vi "DataLoggerModule.vi"(8 "error in (no error)":errorcluster, 9 "Shutdown Event":refnum<user-event>, 10 "Config":cluster{"Tag List":string[]}, 11 "ModuleID":string) -> (0 "error out":errorcluster)   [LabVIEW 2020, in "DataLogger.lvlib"]
uses:
  DataLogger.lvlib
  <vilib>/Tag Engine/Tag/Tag.lvclass
  <vilib>/Tag Engine/Types/SetRequest Cluster.ctl
  <vilib>/Utility/Data Type/Type Definitions/Data Type.ctl
  <vilib>/Tag Engine/Tag/Tag.lvclass/Tag.ctl
  80db7cca-9c65-475a-8561-7a2b6cce7442.vi
  df08592d-67de-40ba-a6cc-0fa837fd12aa.vi
  f9099f2b-b695-4638-8a60-8ed48ec280e8.vi
  5108da9f-c4b3-4642-ad75-afbb112a1f2a.vi
  c28e23b0-67fd-4dd8-8582-f417e2518810.vi
  2954e155-24bd-4d8b-b20f-9ca0e37c8e83.vi
  <vilib>/Tag Engine/Tag/Read Name.vi
  <vilib>/Tag Engine/Tag/Read Units.vi
  <vilib>/Tag Engine/API/Get Tag SetRequest Event.vi
  <vilib>/Tag Engine/Tools/SubVIs/Array of VData to VCluster_openG.vi
  <vilib>/Tag Engine/API/Get Tag Value_ByRef.vi
  <vilib>/Tag Engine/API/Write Tag Value_ByRef.vi
  <vilib>/Tag Engine/Tag/Read SetRequest Event.vi
  <vilib>/Tag Engine/Tag/Read Value.vi
  <vilib>/Tag Engine/Tag/Read Timestamp.vi
  <vilib>/Tag Engine/Tag/Write Value with Timestamp.vi
  <vilib>/Utility/Data Type/Get Type Information.vi
  <vilib>/JDP Science/JSONtext/Variant to JSON Text.vi
  <vilib>/Tag Engine/Core/Tag Lookup_By Name.vi
  <vilib>/Utility/Data Type/Get Cluster Information.vi
  <vilib>/Utility/Data Type/NI_Data Type.lvlib
  <vilib>/Tag Engine/Tag Engine Core.lvlib
  <vilib>/Tag Engine/Tag Engine.lvlib
  1b9bca86-45d1-4ef5-b749-ac0dbadf3a5e.vi
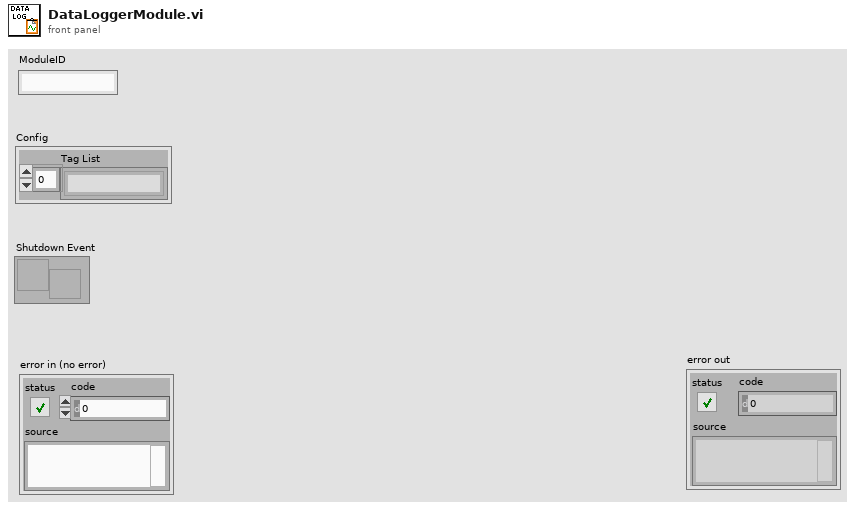
[diagram p1: front panel]
types:
  T1 = cluster{"LOG_EN":refnum<user-event>, "FILE":refnum<user-event>, "PERIOD":refnum<user-event>}
  T2 = cluster{"Tag Refs":cluster{"LOG_EN":refnum<data-value>, "FILE":refnum<data-value>, "PERIOD":refnum<data-value>}, "Config":cluster{"Tag List":string[]}, "LogTagRefs":refnum<data-value>[], "Period":i32, "En":bool, "FileRef":refnum<file>, "FilePath":path}
  T3 = cluster{"LOG_EN":refnum<data-value>, "FILE":refnum<data-value>, "PERIOD":refnum<data-value>}
  T4 = cluster{"Req Value":i32, "Callback":refnum<notifier>}
  T5 = cluster{"Req Value":path, "Callback":refnum<notifier>}
  T6 = enum16{"open", "replace", "create", "open or create", "replace or create", "replace or create with confirmation"}
  T7 = cluster{"Req Value":variant, "Callback":refnum<notifier>}
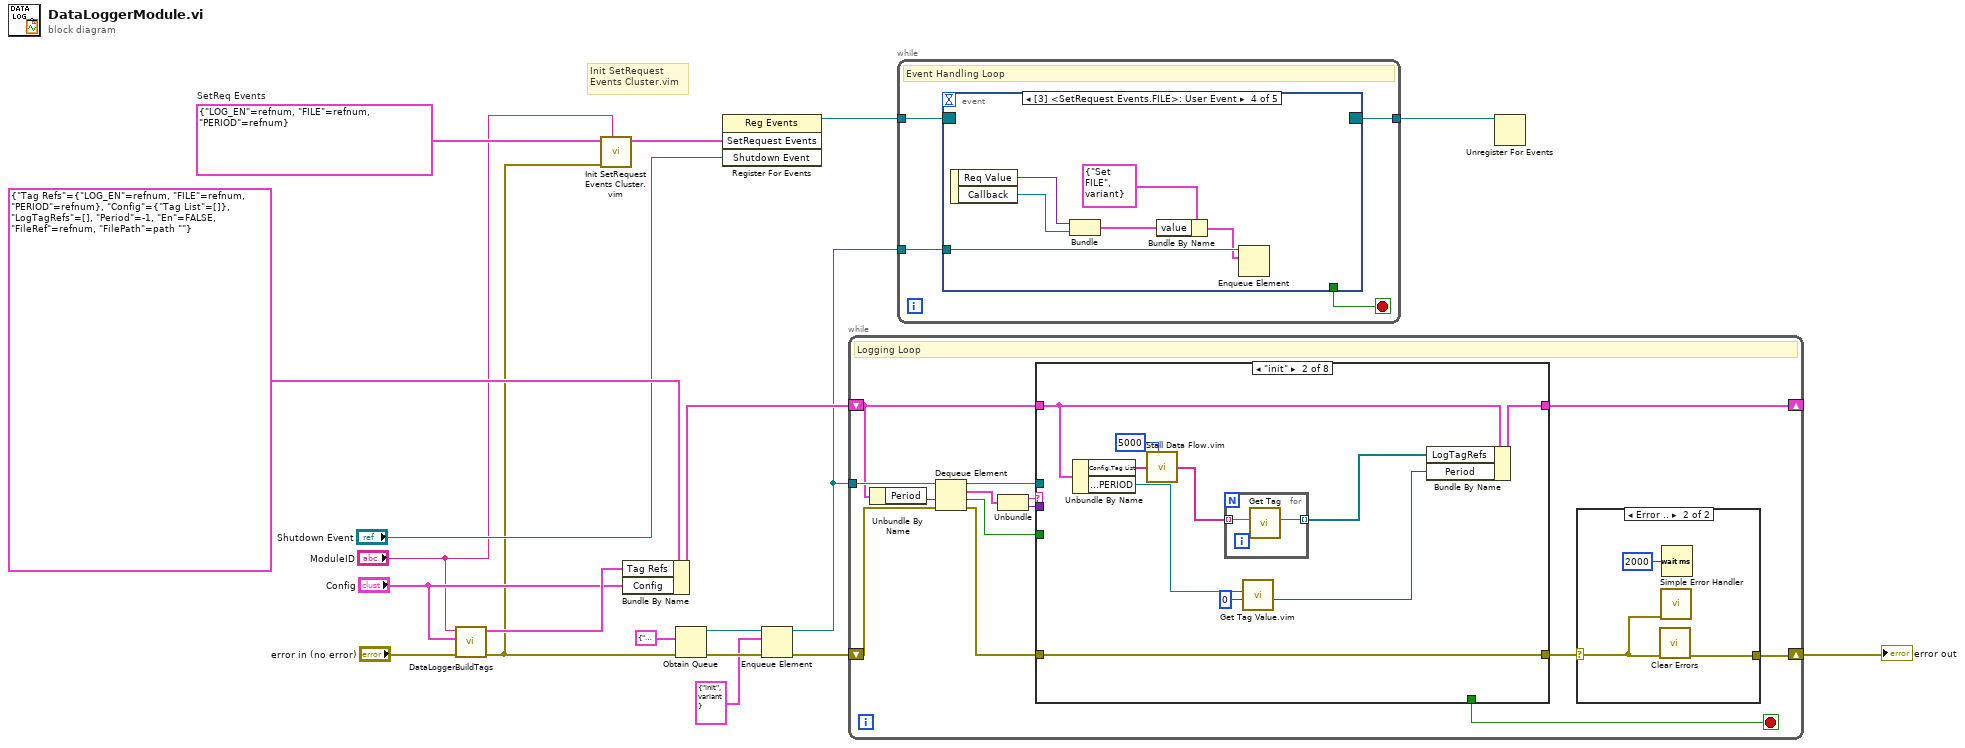
[diagram p0: block diagram]
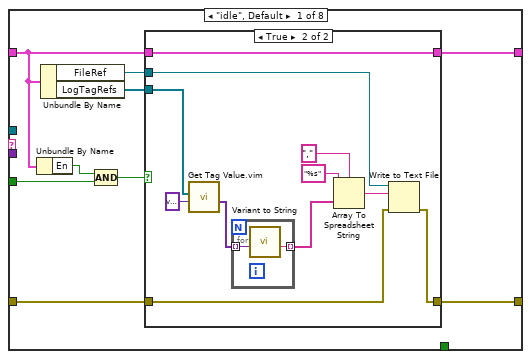
[diagram p3: hidden frame]
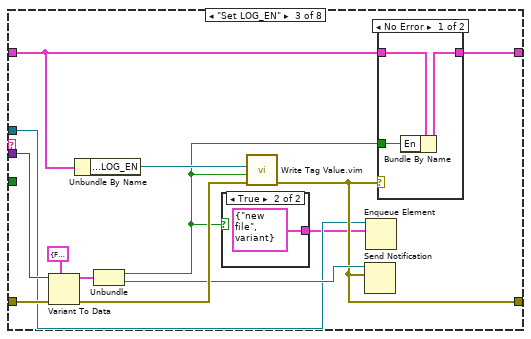
[diagram p5: hidden frame]
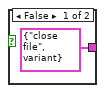
[diagram p6: hidden frame]
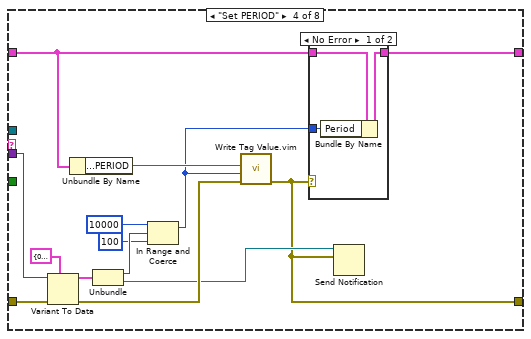
[diagram p8: hidden frame]
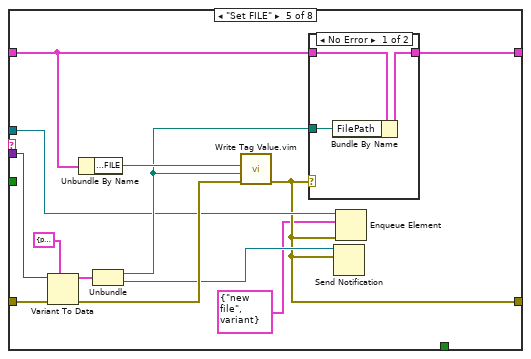
[diagram p10: hidden frame]
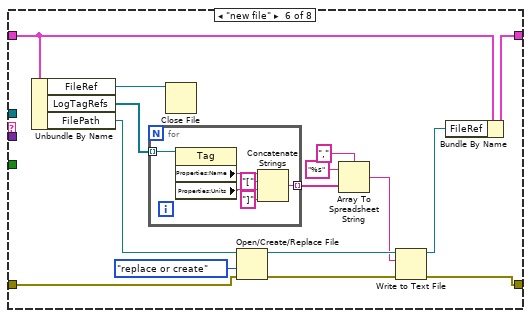
[diagram p12: hidden frame]
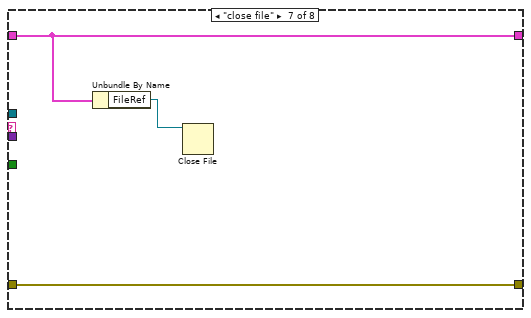
[diagram p13: hidden frame]
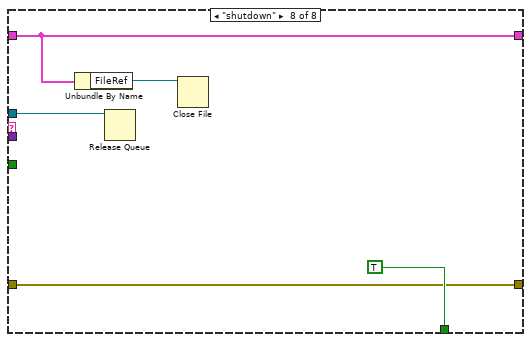
[diagram p14: hidden frame]
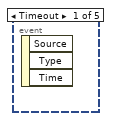
[diagram p15: hidden frame]
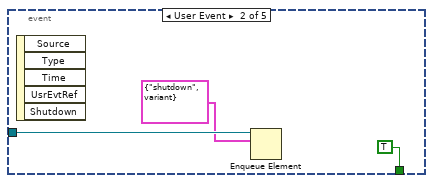
[diagram p16: hidden frame]
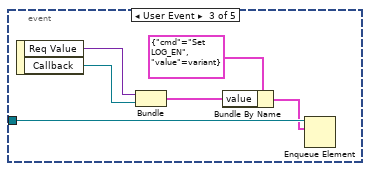
[diagram p17: hidden frame]
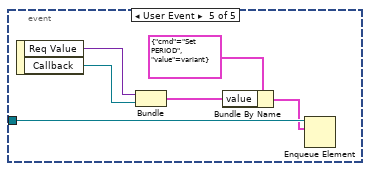
[diagram p18: hidden frame]
diagram:
  w5 = T1 {"LOG_EN"=refnum, "FILE"=refnum, "PERIOD"=refnum}  # SetReq Events
  # "Init SetRequest\nEvents Cluster.vim"
  n1 = call "DataLoggerBuildTags.vi"("error in (no error)"="error in (no error)", "Config"="Config", "ModuleID"="ModuleID") -> ("error out"=w2:errorcluster, "Tag Refs"=w12:T3)  [unwired: 7 in]
  n2 = call "Init SetRequest Events Cluster.vim"("Namespace"="ModuleID", "error in (no error)"=w2, "SetRequest Events in"=w5) -> ("SetRequest Events"=w3:T1)  [unwired: 7 in, 1 out]
  n3 = Bundle By Name(cluster=T2 {"Tag Refs"={"LOG_EN"=refnum, "FILE"=refnum, "PERIOD"=refnum}, "Config"={"Tag List"=[]}, "LogTagRefs"=[], "Period"=-1, "En"=FALSE, "FileRef"=refnum, "FilePath"=path ""}, "Tag Refs"=w12, "Config"="Config") -> (w13:T2)
  n4 = Obtain Queue(element data type=cluster{"cmd":string, "value":variant} {"cmd"="", "value"=variant}, error in (no error)=w2) -> (queue out=w7:refnum<queue>, error out=w10:errorcluster)  [unwired: 3 in, 1 out]
  n5 = register-events(w3, "Shutdown Event") -> (reference out=w19:refnum<event-registration>)  [unwired: 2 in, 1 out]
  n6 = Enqueue Element(queue=w7, element=cluster{"cmd":string, "value":variant} {"cmd"="init", "value"=variant}, error in (no error)=w10) -> (queue out=w8:refnum<queue>, error out=w9:errorcluster)  [unwired: 1 in, 1 out]
  n7 = while {
    tunnel: w8 -> [w33]
    shift-right: [w20] -> w16
    shift-left: w9 -> [w29]
    shift-right: [w26] -> _
    shift-left: w13 -> [w24]
    stop <- w25 stop-if-true
    # "Logging Loop"
    n8 = Unbundle By Name(w24) -> ("Period"=w23:i32)
    n9 = Dequeue Element(queue=w33, timeout in ms (-1)=w23, error in (no error)=w29) -> (queue out=w31:refnum<queue>, element=w32:cluster{"cmd":string, "value":variant}, timed out?=w22:bool, error out=w28:errorcluster)
    n10 = Unbundle(w32) -> ("cmd"=w30:string, "value"=w27:variant)
    n11 = case shown="\"init\"" w30 {
      tunnel: w31 -> [_ _ w75 _ w113 _ _ w156]
      tunnel: w28 -> [w38 w68 w84 w106 w123 w134 w149 w154]
      tunnel: w24 -> [w43 w71 w80 w100 w118 w141 w151 w153]
      tunnel: w27 -> [_ _ w83 w105 w122 _ _ _]
      tunnel: [w39 w68 w77 w93 w112 w129 w149 w154] -> w21
      tunnel: [w40 w69 w82 w103 w120 w140 w151 w153] -> w26
      tunnel: [_ _ _ _ _ _ _ TRUE] -> w25
      tunnel: w22 -> [w45 _ _ _ _ _ _ _]
      frame "idle", Default {
        n12 = Unbundle By Name(w43) -> ("En"=w46:bool)
        n13 = Unbundle By Name(w43) -> ("FileRef"=w41:refnum<file>, "LogTagRefs"=w42:refnum<data-value>[])
        n14 = Compound Arithmetic op=AND(w46, w45) -> (w44:bool)
        n15 = case shown="True" w44 {
          tunnel: w43 -> [w48 w59]
          tunnel: w42 -> [_ w49]
          tunnel: w41 -> [_ w56]
          tunnel: [w48 w59] -> w40
          tunnel: [w47 w54] -> w39
          tunnel: w38 -> [w47 w53]
          frame False {
          }
          frame True {
            n16 = call "Get Tag Value.vim"("Default (Void)"=variant, "Tag Name(s)/Ref(s)"=w49) -> ("Value(s)"=w52:variant[])  [unwired: 6 in, 3 out]
            n17 = for {
              tunnel: w52 -> [w61] mode=indexing
              tunnel: [w60] -> w51 mode=indexing
              n18 = call <vilib>:"Variant to String.vi"("Variant Value"=w61) -> ("String Value"=w60:string)  [unwired: 9 in, 1 out]
            }
            n19 = Array To Spreadsheet String(delimiter (Tab)=",", array=w51, 3:"%s" ("format string")) -> (spreadsheet string=w55:string)
            n20 = Write to Text File(file (use dialog)=w56, text=w55, error in=w53) -> (error out=w54:errorcluster)  [unwired: 1 in, 2 out]
          }
        }
      }
      frame "init" {
        n21 = Unbundle By Name(w71) -> ("Config.Tag List"=w64:string[], "Tag Refs.PERIOD"=w65:refnum<data-value>)
        n22 = call "Stall Data Flow.vim"("value in"=w64, "milliseconds to wait"=u32 5000) -> ("value out"=w63:string[])  [unwired: 1 out]
        n23 = for {
          tunnel: w63 -> [w73] mode=indexing
          tunnel: [w72] -> w70 mode=indexing
          n24 = call <vilib>:"Get Tag.vi"("Name"=w73) -> ("Tag Ref out"=w72:refnum<data-value>)  [unwired: 8 in, 2 out]
        }
        n25 = call "Get Tag Value.vim"("Default (Void)"=0, "Tag Name(s)/Ref(s)"=w65) -> ("Value(s)"=w66:i32)  [unwired: 6 in, 3 out]
        n26 = Bundle By Name(cluster=w71, "LogTagRefs"=w70, "Period"=w66) -> (w69:T2)
      }
      frame "Set LOG_EN" {
        n27 = Variant To Data(error in=w84, type=cluster{bool, "Callback":refnum<notifier>} {FALSE, "Callback"=refnum} ("output cluster"), Variant=w83) -> (data=w85:cluster{bool, "Callback":refnum<notifier>}, error out=w79:errorcluster)
        n28 = Unbundle By Name(w80) -> ("Tag Refs.LOG_EN"=w81:refnum<data-value>)
        n29 = Unbundle(w85) -> (w76:bool, "Callback"=w78:refnum<notifier>)
        n30 = case shown="True" w76 {
          tunnel: [cluster{"cmd":string, "value":variant} {"cmd"="close file", "value"=variant} ("element") cluster{"cmd":string, "value":variant} {"cmd"="new file", "value"=variant} ("element")] -> w74
          frame False {
          }
          frame True {
          }
        }
        n31 = call "Write Tag Value.vim"("error in (no error)"=w79, "Value"=w76, "Tag Name(s)/Ref(s)"=w81) -> ("error out"=w77:errorcluster)  [unwired: 7 in, 1 out]
        n32 = Send Notification(notification=w77, notifier=w78) -> ()  [unwired: 1 in, 2 out]
        n33 = Enqueue Element(queue=w75, element=w74) -> ()  [unwired: 2 in, 3 out]
        n34 = case shown="No Error" w77 {
          tunnel: [w91 w92] -> w82
          tunnel: w80 -> [w90 w92]
          tunnel: w76 -> [w89 _]
          frame No Error {
            n35 = Bundle By Name(cluster=w90, "En"=w89) -> (w91:T2)
          }
          frame Error {
          }
        }
      }
      frame "Set PERIOD" {
        n36 = Variant To Data(error in=w106, type=T4 {"Req Value"=0, "Callback"=refnum} ("output cluster"), Variant=w105) -> (data=w102:T4, error out=w95:errorcluster)
        n37 = Unbundle By Name(w100) -> ("Tag Refs.PERIOD"=w97:refnum<data-value>)
        n38 = Unbundle(w102) -> ("Req Value"=w101:i32, "Callback"=w94:refnum<notifier>)
        n39 = In Range and Coerce(upper limit=10000, x=w101, lower limit=100) -> (coerced(x)=w96:i32)  [unwired: 1 out]
        n40 = call "Write Tag Value.vim"("error in (no error)"=w95, "Value"=w96, "Tag Name(s)/Ref(s)"=w97) -> ("error out"=w93:errorcluster)  [unwired: 7 in, 1 out]
        n41 = case shown="No Error" w93 {
          tunnel: [w109 w110] -> w103
          tunnel: w100 -> [w108 w110]
          tunnel: w96 -> [w107 _]
          frame No Error {
            n42 = Bundle By Name(cluster=w108, "Period"=w107) -> (w109:T2)
          }
          frame Error {
          }
        }
        n43 = Send Notification(notification=w93, notifier=w94) -> ()  [unwired: 1 in, 2 out]
      }
      frame "Set FILE" {
        n44 = Variant To Data(error in=w123, type=T5 {"Req Value"=path "", "Callback"=refnum} ("output cluster"), Variant=w122) -> (data=w119:T5, error out=w116:errorcluster)
        n45 = Unbundle By Name(w118) -> ("Tag Refs.FILE"=w117:refnum<data-value>)
        n46 = Unbundle(w119) -> ("Req Value"=w114:path, "Callback"=w115:refnum<notifier>)
        n47 = call "Write Tag Value.vim"("error in (no error)"=w116, "Value"=w114, "Tag Name(s)/Ref(s)"=w117) -> ("error out"=w112:errorcluster)  [unwired: 7 in, 1 out]
        n48 = case shown="No Error" w112 {
          tunnel: [w126 w127] -> w120
          tunnel: w118 -> [w125 w127]
          tunnel: w114 -> [w124 _]
          frame No Error {
            n49 = Bundle By Name(cluster=w125, "FilePath"=w124) -> (w126:T2)
          }
          frame Error {
          }
        }
        n50 = Send Notification(notification=w112, notifier=w115) -> ()  [unwired: 1 in, 2 out]
        n51 = Enqueue Element(queue=w113, element=cluster{"cmd":string, "value":variant} {"cmd"="new file", "value"=variant}, error in (no error)=w112) -> ()  [unwired: 1 in, 3 out]
      }
      frame "new file" {
        n52 = Unbundle By Name(w141) -> ("FileRef"=w142:refnum<file>, "LogTagRefs"=w139:refnum<data-value>[], "FilePath"=w128:path)
        n53 = for {
          tunnel: w139 -> [w148] mode=indexing
          tunnel: [w143] -> w138 mode=indexing
          n54 = property class="Tag"(reference=w148) -> ("Properties:Name"=w147:string, "Properties:Units"=w145:string)  [unwired: 1 in, 2 out]
          n55 = Concatenate Strings(w147, "[" ("string"), w145, "]" ("string")) -> (w143:string)
        }
        n56 = Close File(refnum=w142) -> ()  [unwired: 1 in, 2 out]
        n57 = Open/Create/Replace File(file path (use dialog)=w128, error in=w134, operation (0:open)=T6."replace or create") -> (refnum out=w132:refnum<file>, error out=w133:errorcluster)  [unwired: 3 in, 1 out]
        n58 = Array To Spreadsheet String(delimiter (Tab)=",", array=w138, 3:"%s" ("format string")) -> (spreadsheet string=w130:string)
        n59 = Write to Text File(file (use dialog)=w132, text=w130, error in=w133) -> (refnum out=w131:refnum<file>, error out=w129:errorcluster)  [unwired: 1 in, 1 out]
        n60 = Bundle By Name(cluster=w141, "FileRef"=w131) -> (w140:T2)
      }
      frame "close file" {
        n61 = Unbundle By Name(w151) -> ("FileRef"=w150:refnum<file>)
        n62 = Close File(refnum=w150) -> ()  [unwired: 1 in, 2 out]
      }
      frame "shutdown" {
        n63 = Unbundle By Name(w153) -> ("FileRef"=w152:refnum<file>)
        n64 = Release Queue(queue=w156) -> ()  [unwired: 2 in, 3 out]
        n65 = Close File(refnum=w152) -> ()  [unwired: 1 in, 2 out]
      }
    }
    n66 = case shown="Error .." w21 {
      selector: w21 -> [w34 w36]
      tunnel: [w34 w35] -> w20
      frame No Error {
      }
      frame Error {
        n67 = call <vilib>:"Clear Errors.vi"("error in (no error)"=w36) -> ("error out"=w35:errorcluster)  [unwired: 5 in, 1 out]
        n68 = call <vilib>:"Simple Error Handler.vi"("error in (no error)"=w36) -> ()  [unwired: 4 in, 5 out]
        n69 = Wait (ms)(milliseconds to wait=u32 2000) -> ()  [unwired: 1 out]
      }
    }
  }
  "error out" <- w16
  n70 = while {
    tunnel: w19 -> [w160]
    tunnel: w8 -> [w158]
    tunnel: [w157] -> w15
    stop <- w159 stop-if-true
    # "Event Handling Loop"
    n71 = event shown="[3] <SetRequest Events.FILE>: User Event" {
      selector: w160 -> [_ _ _ _ _]
      dyn-events: [_ _ _ _ _] -> w157
      timeout: _ -> [_ _ _ _ _]
      tunnel: [_ TRUE _ _ _] -> w159
      tunnel: w158 -> [_ w162 w167 w173 w179]
      event Timeout {
        n72 = event-data() -> ()  [unwired: 1 in, 3 out]
      }
      event User Event {
        n73 = event-data() -> ()  [unwired: 1 in, 5 out]
        n74 = Enqueue Element(queue=w162, element=cluster{"cmd":string, "value":variant} {"cmd"="shutdown", "value"=variant}) -> ()  [unwired: 2 in, 3 out]
      }
      event User Event {
        n75 = event-data() -> ("Req Value"=w169:variant, "Callback"=w168:refnum<notifier>)  [unwired: 1 in]
        n76 = Bundle("Req Value"=w169, "Callback"=w168) -> (w165:T7)  [unwired: 1 in]
        n77 = Bundle By Name(cluster=cluster{"cmd":string, "value":variant} {"cmd"="Set LOG_EN", "value"=variant} ("element"), "value"=w165) -> (w164:cluster{"cmd":string, "value":variant})
        n78 = Enqueue Element(queue=w167, element=w164) -> ()  [unwired: 2 in, 3 out]
      }
      event User Event {
        n79 = event-data() -> ("Req Value"=w175:variant, "Callback"=w174:refnum<notifier>)  [unwired: 1 in]
        n80 = Bundle("Req Value"=w175, "Callback"=w174) -> (w171:T7)  [unwired: 1 in]
        n81 = Bundle By Name(cluster=cluster{"cmd":string, "value":variant} {"cmd"="Set FILE", "value"=variant} ("element"), "value"=w171) -> (w170:cluster{"cmd":string, "value":variant})
        n82 = Enqueue Element(queue=w173, element=w170) -> ()  [unwired: 2 in, 3 out]
      }
      event User Event {
        n83 = event-data() -> ("Req Value"=w181:variant, "Callback"=w180:refnum<notifier>)  [unwired: 1 in]
        n84 = Bundle("Req Value"=w181, "Callback"=w180) -> (w177:T7)  [unwired: 1 in]
        n85 = Bundle By Name(cluster=cluster{"cmd":string, "value":variant} {"cmd"="Set PERIOD", "value"=variant} ("element"), "value"=w177) -> (w176:cluster{"cmd":string, "value":variant})
        n86 = Enqueue Element(queue=w179, element=w176) -> ()  [unwired: 2 in, 3 out]
      }
    }
  }
  n87 = Unregister For Events(event registration refnum=w15) -> ()  [unwired: 1 in, 1 out]
